vi "E727_Sample_Application_With_Analog.vi"() -> ()   [LabVIEW 2014]
doc: "This VI demonstrates the use of digital (e.g. RS-232) communication and analog interfacing in parallel for the E-727. In this example the E-727 is connected through COM port 1 with baudrate 115200. The VI first initializes the E-727 via the selected digital interface by running E727_Configuration_Setup.vi . It then switches to analog control, using SwitchToAnalogOrDigital.vi and initializes the analog interface by running Analog_Configuration_Setup.vi . After these initialization steps, it moves one axis relative to its current position by outputting a voltage by the DAC card used, waits 10 ms and queries for the position of this axis. Finally, it switches back to digital control and closes both the analog and the digital connection to the controller. \nAs the E-727 provides no Sensor Monitor Output, connect the Analog Out line of the DAC card to the corresponding Analog In line of the card. \nThe diagram shows how to combine the driver VIs for these tasks. \nWarning: Before running this VI, modify the \"Interface\" and \"RS232 settings\" (or TCP/IP settings or USB settings ) to reflect your configuration. The predefined settings provided with the VI probably do not match your system."
panel:
  out "Running 2":bool caption="Analog_Configuration_Setup.vi is running"
  in  "stop":bool
  in  "error in":errorcluster
  out "Running":bool caption="E727_Configuration_Setup.vi is running"
  out "error out":errorcluster
  out "Position":dbl[](array[numeric]) format="%.6f"
  out "Conn. Axis":string[](array[string])
  out "E-727 Identification":string
  # "This This VI demonstrates the use of digital (e.g. RS-232) communication and analog interfacing in parallel for the E-727.  The diagram\nshows how to combine the driver VIs for these tasks.\n\nWarning: Before running this VI, modify the interface settings on the block diagram to reflect your configuration. The predefined \n                 settings provided with the VI probably do not match your system.\n                 Both the E-727 Digital LabVIEW driver set and the GCS Analog LabVIEW driver set must be installed, otherwise the VI will not\n                 be executable."
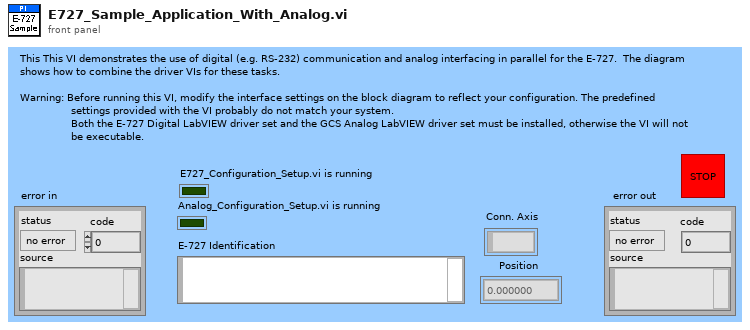
[diagram p1: front panel]
types:
  T1 = cluster{"Conn. Axes":string[], "AI channels":tag[], "AO channels":tag[], "Lower voltage limit (V)":dbl, "Upper voltage limit (V)":dbl, "AI Sample Rate":dbl, "AI Samples/Channel":i32}
  T2 = cluster{"Host address/name":string, "Port":i32, "Board":i32, "TCP/IP Search?":bool}
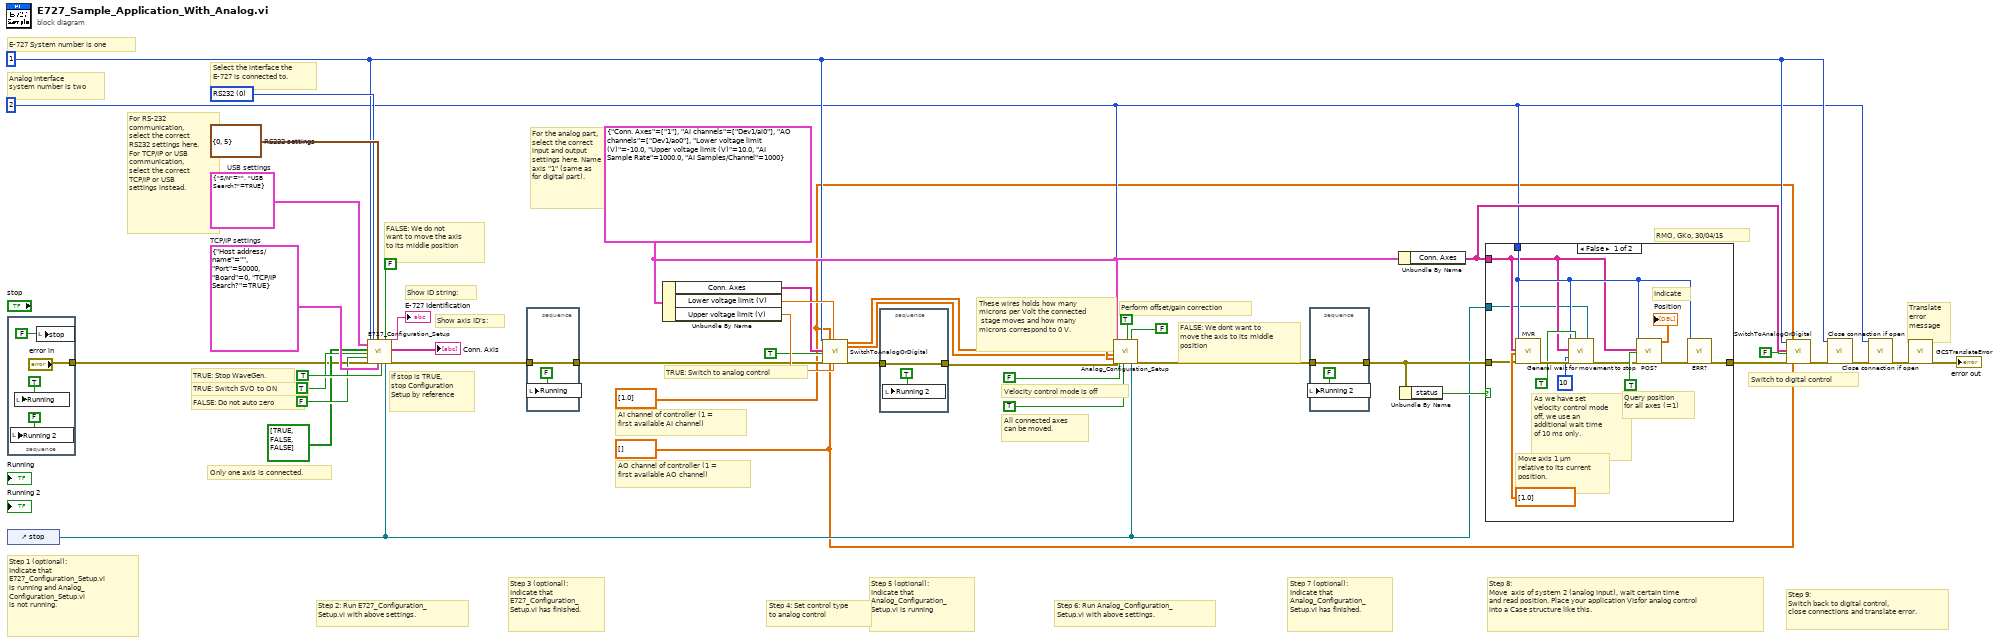
[diagram p0: block diagram]
diagram:
  w1 = dbl[] [] ("AO channels")
  w2 = dbl[] [1.0] ("AI channels")
  w20 = T1 {"Conn. Axes"=["1"], "AI channels"=["Dev1/ai0"], "AO channels"=["Dev1/ao0"], "Lower voltage limit (V)"=-10.0, "Upper voltage limit (V)"=10.0, "AI Sample Rate"=1000.0, "AI Samples/Channel"=1000} ("Input/output settings")
  w4 = 2 ("System no.")
  w26 = cluster{"S/N":string, "USB Search?":bool} {"S/N"="", "USB Search?"=TRUE}  # USB settings
  w32 = u16 0 items=["RS232", "TCP/IP", "USB"] ("Interface")
  w34 = cluster{"Portnumber":i32, "Baudrate":u16} {"Portnumber"=0, "Baudrate"=5}  # RS232 settings
  w39 = T2 {"Host address/name"="", "Port"=50000, "Board"=0, "TCP/IP Search?"=TRUE}  # TCP/IP settings
  w5 = 1 ("System no.")
  # "RMO, GKo, 30/04/15"
  # "Step 7 (optional):\nIndicate that\nAnalog_Configuration_\nSetup.vi has finished."
  # "Step 5 (optional):\nIndicate that\nAnalog_Configuration_\nSetup.vi is running"
  # "Step 3 (optional):\nIndicate that\nE727_Configuration_\nSetup.vi has finished."
  # "Step 4: Set control type\nto analog control"
  # "Step 9: \nSwitch back to digital control,\nclose connections and translate error."
  # "Translate\nerror \nmessage"
  # "Switch to digital control"
  # "AO channel of controller (1 = \nfirst available AO channel)"
  # "AI channel of controller (1 = \nfirst available AI channel)"
  # "TRUE: Switch to analog control"
  # "Step 6: Run Analog_Configuration_\nSetup.vi with above settings."
  # "Velocity control mode is off"
  # "FALSE: We dont want to\nmove the axis to its middle\nposition"
  # "Perform offset/gain correction"
  # "All connected axes\ncan be moved."
  # "These wires holds how many\nmicrons per Volt the connected\n stage moves and how many\nmicrons correspond to 0 V."
  # "For the analog part,\nselect the correct\ninput and output \nsettings here. Name\naxis \"1\" (same as \nfor digital part)."
  # "Analog interface \nsystem number is two"
  # "Only one axis is connected."
  # "FALSE: We do not\nwant to move the axis\nto its middle position"
  # "FALSE: Do not auto zero"
  # "TRUE: Switch SVO to ON"
  # "If stop is TRUE, \nstop Configuration\nSetup by reference"
  # "Step 8: \nMove  axis of system 2 (analog input), wait certain time\nand read position. Place your application VIsfor analog control\ninto a Case structure like this."
  # "For RS-232 \ncommunication,\nselect the correct\nRS232 settings here.\nFor TCP/IP or USB \ncommunication, \nselect the correct \nTCP/IP or USB\nsettings instead."
  # "Select the interface the \nE-727 is connected to."
  # "Step 2: Run E727_Configuration_\nSetup.vi with above settings."
  # "Step 1 (optional): \nIndicate that\nE727_Configuration_Setup.vi\nis running and Analog_\nConfiguration_Setup.vi\nis not running."
  # "Show axis ID's:"
  # "Show ID string:"
  # "TRUE: Stop WaveGen."
  # "E-727 System number is one"
  n1 = stacked-sequence {
    tunnel: ["error in"] -> w13
    frame #0 {
      n2 = local write "Running 2"(FALSE ("Running")) -> ()
      n3 = local write "Running"(TRUE ("Running")) -> ()
      n4 = local write "stop"(FALSE ("stop")) -> ()
    }
  }
  n5 = control-ref of="stop"() -> (w14:refnum<vi>)
  n6 = call "E727_Configuration_Setup.vi"("System no."=w5, "USB settings"=w26, "Are stages connected?"=bool[] [TRUE, FALSE, FALSE], "Change servo status to ON?"=TRUE ("Use dialog to define\nconnected stages?"), "Perform autozero?"=FALSE ("Use dialog to define\nconnected stages?"), "error in"=w13, "Interface"=w32, "RS232 settings"=w34, "TCP/IP settings"=w39, "Stop wave generator\noutput (if any)"=TRUE ("All axes?"), "Move to middle?"=FALSE, "Stop refnum"=w14) -> ("Identification"=→"E-727 Identification":string, "All conn. axes"=→"Conn. Axis":string[], "error out"=w9:errorcluster)  [unwired: 2 in, 3 out]
  n7 = stacked-sequence {
    tunnel: w9 -> [w48]
    tunnel: [w48] -> w10
    frame #0 {
      n8 = local write "Running"(FALSE ("Running")) -> ()
    }
  }
  n9 = Unbundle By Name(w20) -> ("Conn. Axes"=w17:string[], "Lower voltage limit (V)"=w25:dbl, "Upper voltage limit (V)"=w24:dbl)
  n10 = call "SwitchToAnalogOrDigital.vi"("System no."=w5, "Axes to command"=w17, "Mode"=TRUE ("Mode (Analog: T)"), "error in"=w10, "AI channels"=w2, "AO channels"=w1, "Lower voltage limit (V)"=w25, "Upper voltage limit (V)"=w24) -> ("Conversion factor"=w22:dbl[], "Offset"=w3:dbl[], "Error out"=w12:errorcluster)  [unwired: 3 in, 6 out]
  n11 = stacked-sequence {
    tunnel: [w49] -> w11
    tunnel: w12 -> [w49]
    frame #0 {
      n12 = local write "Running 2"(TRUE ("Running")) -> ()
    }
  }
  n13 = call "Analog_Configuration_Setup.vi"("System no."=w4, "Input/output settings"=w20, "Conversion offset"=w3, "Conversion factor"=w22, "error in"=w11, "Vel. control mode"=FALSE, "All axes?"=TRUE, "Offset/Gain\ncorrection"=TRUE ("Offset/Gain\ncorrection"), "Move \nto middle?"=FALSE ("Move \nto middle?"), "Stop refnum"=w14) -> ("error out"=w31:errorcluster)  [unwired: 3 in, 6 out]
  n14 = stacked-sequence {
    tunnel: w31 -> [w52]
    tunnel: [w52] -> w41
    frame #0 {
      n15 = local write "Running 2"(FALSE ("Running")) -> ()
    }
  }
  n16 = Unbundle By Name(w20) -> ("Conn. Axes"=w16:string[])
  n17 = Unbundle By Name(w41) -> ("status"=w40:bool)
  n18 = case shown="False" w40 {
    tunnel: [w53 w66] -> w18
    tunnel: w41 -> [w56 w66]
    tunnel: w14 -> [w54 _]
    tunnel: w4 -> [w58 _]
    tunnel: w16 -> [w55 _]
    frame False {
      # "As we have set\nvelocity control mode\noff, we use an\nadditional wait time\nof 10 ms only."
      # "Indicate"
      # "Query position\nfor all axes (=1)"
      # "Move axis 1 µm\nrelative to its current\nposition."
      n19 = call "MVR.vi"("System no."=w58, "Axes to move"=w55, "Position values"=dbl[] [1.0], "error in"=w56) -> ("error out"=w63:errorcluster)  [unwired: 1 in, 14 out]
      n20 = call "General wait for movement to stop.vi"("System no."=w58, "Axes to wait for"=w55, "Additional wait time, ms"=u32 10, "error in"=w63, "Add. wait only?"=TRUE, "Stop refnum"=w54) -> ("error out"=w62:errorcluster)  [unwired: 2 in, 11 out]
      n21 = call "POS?.vi"("System no."=w58, "Axes to query"=w55, "All axes?"=TRUE, "error in"=w62) -> ("Position"=→"Position":dbl[], "error out"=w61:errorcluster)  [unwired: 1 in, 13 out]
      n22 = call "ERR?.vi"("System no."=w58, "error in"=w61) -> ("error out"=w53:errorcluster)  [unwired: 17 out]
    }
    frame True {
      # "Error during initialization"
    }
  }
  n23 = call "SwitchToAnalogOrDigital.vi"("System no."=w5, "Axes to command"=w16, "Mode"=FALSE, "error in"=w18, "AI channels"=w2, "AO channels"=w1) -> ("Error out"=w8:errorcluster)  [unwired: 3 in, 10 out]
  n24 = call "Close connection if open.vi"("System no."=w5, "error in"=w8) -> ("error out"=w7:errorcluster)  [unwired: 1 in, 16 out]
  n25 = call "Close connection if open.vi"("System no."=w4, "error in"=w7) -> ("error out"=w6:errorcluster)  [unwired: 1 in, 16 out]
  n26 = call "GCSTranslateError.vi"("error in"=w6) -> ("error out"=→"error out":errorcluster)  [unwired: 18 out]
